vi "WPI_Power Get 6Volt Rail Voltage and Current.vi"(11 "error in":errorcluster) -> (6 "6 volt rail voltage (V)":dbl, 8 "6 volt rail current (A)":dbl, 15 "error out":errorcluster)   [LabVIEW 2017]
doc: "Returns the voltage and current of the 6 volt user rail on the roboRIO in the robot program. On the roboRIO the 6 volt rail is connected to pin V of PWM channels."
uses:
  <vilib>/Utility/error.llb/Error Cluster From Error Code.vi
  <vilib>/rvi/errors/niLvFpgaAdjustHostInterfaceError.vi
  <vilib>/rvi/interface/nirviReadWriteControl/nirviReadWriteControl.xnode
  <vilib>/Rock Robotics/SystemInterfaces/System/FPGA_SystemFRC FPGA Ref.ctl
  NiFpgaLv.dll
  <vilib>/rvi/interface/Simulation/niFpgaSimulationCallBeginRW.vi
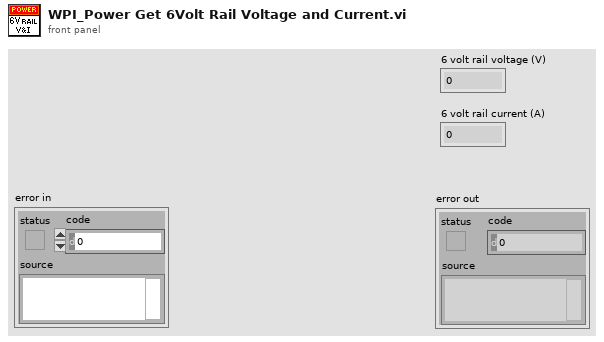
[diagram p1: front panel]
types:
  T1 = typedef "FPGA_SystemFRC FPGA Ref.ctl" = refnum<k20>
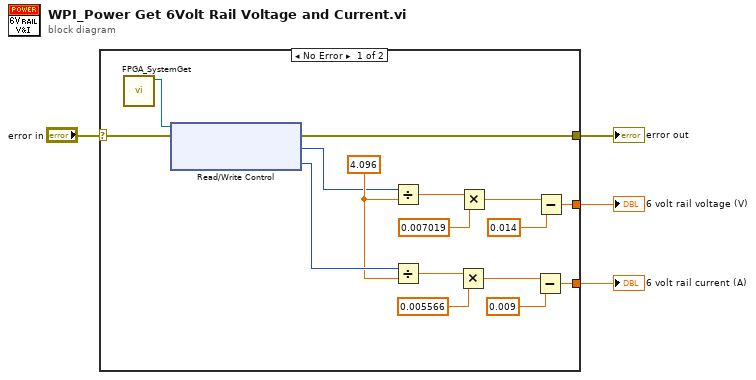
[diagram p0: block diagram]
diagram:
  n1 = case shown="No Error" "error in" {
    selector: "error in" -> [w5 w21]
    tunnel: [w6 w21] -> w3
    tunnel: [w17 _] -> w2
    tunnel: [w13 _] -> w1
    frame No Error {
      w11 = 4.096 ("battery voltage out")
      n2 = call <vilib>:"FPGA_SystemGet.vi"() -> ("FRC FPGA Ref"=w10:T1)  [unwired: 2 in, 9 out]
      n3 = xnode "Read/Write Control"("FPGA VI Reference In"=w10, "error in"=w5) -> ("error out"=w6:errorcluster, "Power.UserVoltage6V"=w9:u16, "Power.UserCurrent6V"=w12:u16)  [unwired: 1 out]
      n4 = Divide(x=w9, y=w11) -> (x/y=w7:dbl)
      n5 = Divide(x=w12, y=w11) -> (x/y=w8:dbl)
      n6 = Multiply(x=w8, y=0.005566 ("battery voltage out")) -> (x*y=w15:dbl)
      n7 = Multiply(x=w7, y=0.007019 ("battery voltage out")) -> (x*y=w19:dbl)
      n8 = Subtract(x=w15, y=0.009 ("battery voltage out")) -> (x-y=w13:dbl)
      n9 = Subtract(x=w19, y=0.014 ("battery voltage out")) -> (x-y=w17:dbl)
    }
    frame Error {
    }
  }
  "error out" <- w3
  "6 volt rail voltage (V)" <- w2
  "6 volt rail current (A)" <- w1
